vi "Pre Launch Init.vi"(11 "Study Actor in":refnum<class "Study Actor.lvclass">) -> (0 "error out":errorcluster, 3 "Study Actor out":refnum<class "Study Actor.lvclass">)   [LabVIEW 2024, in "Study Actor.lvlib" / "Study Actor.lvclass"]
doc: "Initializes the panel actor. Creates the Panel Helper.\n\n----\nPlease see the following web address for additional documentation and tutorial information:\nhttp://www.mooregoodideas.com/mgi-panel-manager/\n\nAuthor: Derek Trepanier\n\nCopyright (c) 2018, Moore Good Ideas, Inc.\n\nAll rights reserved.\n\nRedistribution and use in source and binary forms, with or without modification, are permitted provided that the following conditions are met:\n\n * Redistributions of source code must retain the above copyright notice, this list of conditions and the following disclaimer.\n * Redistributions in binary form must reproduce the above copyright notice, this list of conditions and the following disclaimer in the documentation and/or other materials provided with the distribution.\n * Neither the name of Moore Good Ideas, Inc. nor the names of its contributors may be used to endorse or promote products derived from this software without specific prior written permission.\n\nTHIS SOFTWARE IS PROVIDED BY THE COPYRIGHT HOLDERS AND CONTRIBUTORS \"AS IS\" AND ANY EXPRESS OR IMPLIED WARRANTIES, INCLUDING, BUT NOT LIMITED TO, THE IMPLIED WARRANTIES OF MERCHANTABILITY AND FITNESS FOR A PARTICULAR PURPOSE ARE DISCLAIMED. IN NO EVENT SHALL THE COPYRIGHT OWNER OR CONTRIBUTORS BE LIABLE FOR ANY DIRECT, INDIRECT, INCIDENTAL, SPECIAL, EXEMPLARY, OR CONSEQUENTIAL DAMAGES (INCLUDING, BUT NOT LIMITED TO, PROCUREMENT OF SUBSTITUTE GOODS OR SERVICES; LOSS OF USE, DATA, OR PROFITS; OR BUSINESS INTERRUPTION) HOWEVER CAUSED AND ON ANY THEORY OF LIABILITY, WHETHER IN CONTRACT, STRICT LIABILITY, OR TORT (INCLUDING NEGLIGENCE OR OTHERWISE) ARISING IN ANY WAY OUT OF THE USE OF THIS SOFTWARE, EVEN IF ADVISED OF THE POSSIBILITY OF SUCH DAMAGE."
uses:
  Study Actor.lvclass
  <vilib>/ni/Actors/Network Endpoint Actors/Protocols/Network Stream Strategy/Network Stream/Network Stream.lvclass
  Study Actor.lvclass/Study Actor.ctl
  <vilib>/ni/Actors/Network Endpoint Actors/Protocols/Network Stream Strategy/Network Stream/Network Stream.lvclass/Network Stream.ctl
  <vilib>/MGI/Panel Manager/Panel Actor/Panel Actor/Panel Actor.lvclass
  Reply-Msg-DataSocket/Reply Msg DataSocket/Reply Msg DataSocket.lvclass
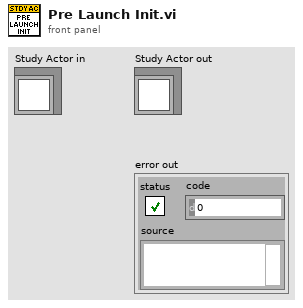
[diagram p1: front panel]
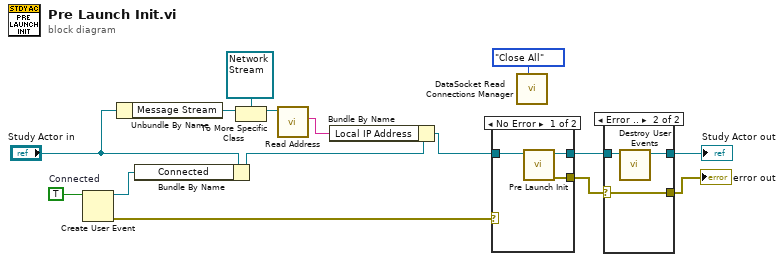
[diagram p0: block diagram]
diagram:
  w15 = TRUE  # Connected
  n1 = Create User Event(user event datatype=w15) -> (user event=w14:refnum<user-event>, error out=w9:errorcluster)  [unwired: 1 in]
  n2 = Unbundle By Name("Study Actor in") -> ("Message Stream"=w5:refnum<class "Message Stream.lvclass">)
  n3 = Bundle By Name(cluster="Study Actor in", "Connected"=w14) -> (w3:refnum<class "Study Actor.lvclass">)
  n4 = To More Specific Class(target class=refnum<class "Network Stream.lvclass"> refnum ("Network Stream in"), reference=w5) -> (specific class reference=w7:refnum<class "Network Stream.lvclass">)  [unwired: 1 in, 1 out]
  n5 = call <vilib>:"Read Address.vi"("Network Stream in"=w7) -> ("Address"=w1:string)  [unwired: 10 in]
  n6 = Bundle By Name(cluster=w3, "Local IP Address"=w1) -> (w2:refnum<class "Study Actor.lvclass">)
  n7 = case shown="No Error" w9 {
    selector: w9 -> [_ w19]
    tunnel: [w18 w19] -> w11
    tunnel: [w17 w20] -> w13
    tunnel: w2 -> [w16 w20]
    frame No Error {
      n8 = call-parent "Pre Launch Init.vi"("Panel Actor in"=w16) -> ("error out"=w18:errorcluster, "Panel Actor out"=w17:refnum<class "Study Actor.lvclass">)  [unwired: 9 in]
    }
    frame Error {
    }
  }
  n9 = call "DataSocket Read Connections Manager.vi"("Action"=enum16{"Get", "Close", "Close All"}."Close All") -> ()  [unwired: 10 in, 1 out]
  n10 = case shown="Error .." w11 {
    selector: w11 -> [w22 w24]
    tunnel: w13 -> [w21 w25]
    tunnel: [w21 w23] -> w12
    tunnel: [w22 w24] -> w10
    frame No Error {
    }
    frame Error {
      n11 = call "Destroy User Events.vi"("Study Actor in"=w25) -> ("Study Actor out"=w23:refnum<class "Study Actor.lvclass">)  [unwired: 10 in]
    }
  }
  "error out" <- w10
  "Study Actor out" <- w12
